vi "velocitymode_read_write_ADC_DAC.vi"() -> ()   [LabVIEW 2018]
uses:
  <vilib>/FPGAPlugInAG/myRIO-1900/niLvFpga_Open_myRIO-1900.vi
  <vilib>/rvi/interface/common/dynamic/niFpgaDynamicAddResources.vi
  <vilib>/Utility/error.llb/Error Cluster From Error Code.vi
  <vilib>/rvi/errors/niLvFpgaAdjustHostInterfaceError.vi
  <vilib>/FPGAPlugInAG/Dynamic/niLvFpga_Close_Dynamic.vi
  <vilib>/rvi/interface/nirviOpenFPGA/nirviOpenFPGA.xnode
  FPGA Bitfiles/WattBalanceRev1_FPGATarget_FPGASPI2_21rs6YSGst0.lvbitx
  FPGA files/FPGA_SPI.vi
  <vilib>/rvi/interface/nirviReadWriteControl/nirviReadWriteControl.xnode
  <vilib>/rvi/interface/nirviCloseFPGA/nirviCloseFPGA.xnode
  NiFpgaLv.dll
  <vilib>/rvi/interface/Simulation/niFpgaSimulationCallBeginRW.vi
panel:
  in  "no. moving avg.":i32=5
  in  "offset (mV)":dbl
  in  "amplitude (V)":dbl
  in  "frequency (Hz)":dbl
  in  "CH1":bool[](array[boolean])=[FALSE, FALSE, TRUE, FALSE, FALSE, TRUE, FALSE, FALSE, FALSE, FALSE, FALSE, FALSE, FALSE, FALSE, FALSE, FALSE]
  in  "CH2":bool[](array[boolean])=[FALSE, FALSE, FALSE, FALSE, FALSE, TRUE, FALSE, FALSE, FALSE, FALSE, FALSE, FALSE, FALSE, FALSE, FALSE, FALSE]
  out "EMF (Velocity mode)":dbl(graph)
  out "Cap probe":dbl(graph)=0.00030517112470818
  in  "Color Box":u32(colorbox)
  in  "stop":bool
  out "avg. loop rate (kHz)":dbl format="%#_2g"
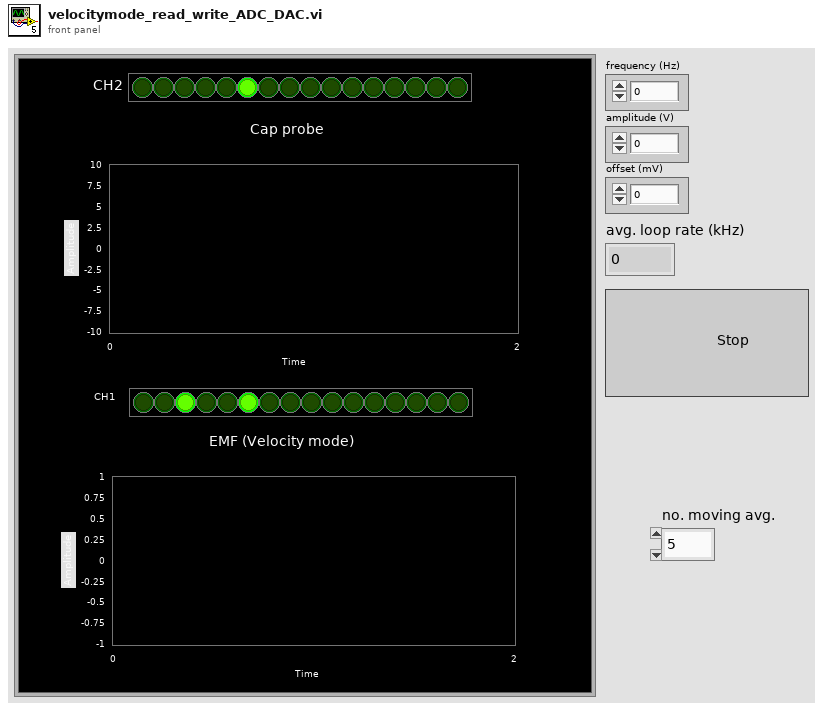
[diagram p1: front panel]
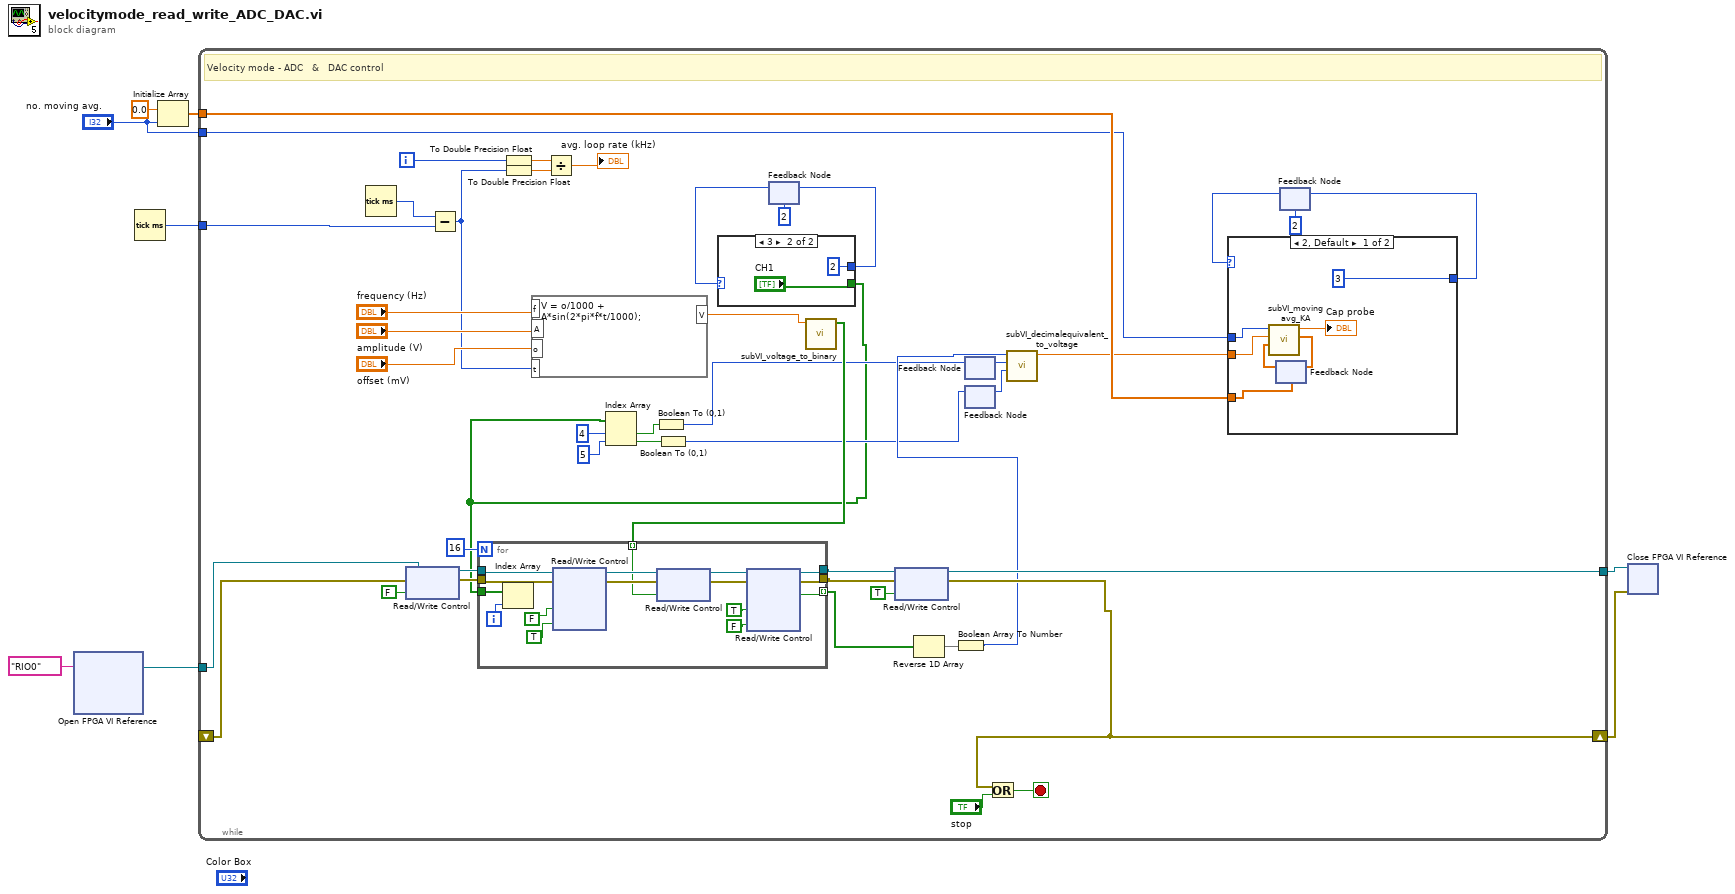
[diagram p0: block diagram]
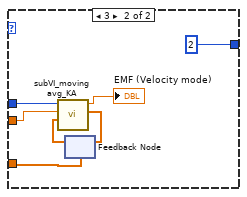
[diagram p2: hidden frame]
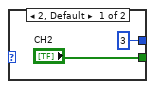
[diagram p3: hidden frame]
diagram:
  n1 = xnode "Open FPGA VI Reference"("resource name"=tag "RIO0") -> ("FPGA VI Reference Out"=w3:refnum<k20>)  [unwired: 1 in, 1 out]
  n2 = Tick Count (ms)() -> (millisecond timer value=w8:u32)
  n3 = Initialize Array(0.0 ("element"), "no. moving avg.") -> (w5:dbl[])
  n4 = while {
    shift-right: [w20] -> w1
    shift-left: _ -> [w21]
    tunnel: w8 -> [w52]
    tunnel: "no. moving avg." -> [w34]
    tunnel: w5 -> [w35]
    tunnel: w3 -> [w22]
    tunnel: [w18] -> w2
    i -> [w41]
    stop <- w53 stop-if-true
    # "Velocity mode - ADC   &   DAC control"
    n5 = Tick Count (ms)() -> (millisecond timer value=w51:u32)
    n6 = xnode "Read/Write Control"("FPGA VI Reference In"=w22, "error in"=w21, "CS"=FALSE) -> ("FPGA VI Reference Out"=w29:refnum<k20>, "error out"=w28:errorcluster)
    n7 = Subtract(x=w51, y=w52) -> (x-y=w37:u32)
    n8 = To Double Precision Float(number=w41) -> (double precision float=w42:dbl)
    n9 = To Double Precision Float(number=w37) -> (double precision float=w43:dbl)
    n10 = formula code="V = o/1000 + \nA*sin(2*pi*f*t/1000);"("f"="frequency (Hz)", "A"="amplitude (V)", "t"=w37, "o"="offset (mV)") -> ("V"=w44:dbl)
    n11 = Divide(x=w42, y=w43) -> (x/y=→"avg. loop rate (kHz)":dbl)
    n12 = feedback #1(2) -> (w49:i32)
    n13 = case shown="3" w49 {
      tunnel: ["CH2" "CH1"] -> w10
      tunnel: [3 2] -> w36
      frame 2, Default {
      }
      frame 3 {
      }
    }
    n14 = Index Array(array=w10, index #1=4 ("index"), index #2=5 ("index")) -> (element #1=w12:bool, element #2=w11:bool)
    n15 = Boolean To (0,1)(Boolean=w12) -> (0, 1=w13:i16)
    n16 = Boolean To (0,1)(Boolean=w11) -> (0, 1=w14:i16)
    n17 = feedback-in #1(w36) -> ()
    n18 = call "subVI_voltage_to_binary.vi"("voltage"=w44) -> ("binary"=w19:bool[])  [unwired: 10 in]
    n19 = for {
      N: 16 -> [_]
      tunnel: w29 -> [w62]
      tunnel: w28 -> [w61]
      tunnel: [w59] -> w24 mode=indexing
      tunnel: [w58] -> w31
      tunnel: [w57] -> w30
      tunnel: w10 -> [w55]
      tunnel: w19 -> [w56] mode=indexing
      i -> [w60]
      n20 = Index Array(array=w55, index=w60) -> ()  [unwired: 1 out]
      n21 = xnode "Read/Write Control"("FPGA VI Reference In"=w62, "error in"=w61, "CLK2"=FALSE ("CLK"), "CLK1"=TRUE ("CLK")) -> ("FPGA VI Reference Out"=w68:refnum<k20>, "error out"=w67:errorcluster)  [unwired: 1 in]
      n22 = xnode "Read/Write Control"("FPGA VI Reference In"=w68, "error in"=w67, "MOSI2"=w56) -> ("FPGA VI Reference Out"=w66:refnum<k20>, "error out"=w65:errorcluster)
      n23 = xnode "Read/Write Control"("FPGA VI Reference In"=w66, "error in"=w65, "CLK2"=TRUE, "CLK1"=FALSE) -> ("FPGA VI Reference Out"=w58:refnum<k20>, "error out"=w57:errorcluster, "MISO1"=w59:bool)
    }
    n24 = xnode "Read/Write Control"("FPGA VI Reference In"=w31, "error in"=w30, "CS"=TRUE) -> ("FPGA VI Reference Out"=w18:refnum<k20>, "error out"=w20:errorcluster)
    n25 = Reverse 1D Array(array=w24) -> (reversed array=w23:bool[])
    n26 = Boolean Array To Number(Boolean array=w23) -> (number=w17:u32)
    n27 = feedback-in #2(w13) -> ()
    n28 = feedback #2() -> (w16:i16)  [unwired: 1 in]
    n29 = feedback #3() -> (w15:i16)  [unwired: 1 in]
    n30 = feedback-in #3(w14) -> ()
    n31 = Or(x=w20, y="stop") -> (x .or. y?=w53:bool)
    n32 = call "subVI_decimalequivalent_to_voltage.vi"("i"=w15, "GAIN"=w16, "UNI"=w17) -> ("V"=w9:dbl)  [unwired: 8 in]
    n33 = feedback #4(2) -> (w46:i32)
    n34 = case shown="2, Default" w46 {
      tunnel: [3 2] -> w47
      tunnel: w9 -> [w71 w78]
      tunnel: w35 -> [w73 w80]
      tunnel: w34 -> [w74 w79]
      frame 2, Default {
        n35 = feedback #5(w73) -> (w75:dbl[])
        n36 = call "subVI_moving avg_KA.vi"("input array"=w75, "sample"=w71, "no. moving avg."=w74) -> ("output array"=w76:dbl[], "avg."=→"Cap probe":dbl)  [unwired: 7 in]
        n37 = feedback-in #5(w76) -> ()
      }
      frame 3 {
        n38 = feedback #6(w80) -> (w83:dbl[])
        n39 = call "subVI_moving avg_KA.vi"("input array"=w83, "sample"=w78, "no. moving avg."=w79) -> ("output array"=w82:dbl[], "avg."=→"EMF (Velocity mode)":dbl)  [unwired: 7 in]
        n40 = feedback-in #6(w82) -> ()
      }
    }
    n41 = feedback-in #4(w47) -> ()
  }
  n42 = xnode "Close FPGA VI Reference"("FPGA VI Reference In"=w2, "error in"=w1) -> ()  [unwired: 1 out]
